vi "list_items.vi"(8 "error in (no error)":errorcluster, 11 "Table in":refnum<class "Table.lvclass">) -> (0 "error out":errorcluster, 2 "items":string[](array[string]), 3 "Table out":refnum<class "Table.lvclass">)   [LabVIEW 2020, in "toml_edit.lvlib" / "Table.lvclass"]
uses:
  Table.lvclass
  Table.lvclass/Table.ctl
  toml_edit.lvlib
  dragon_toml_64.dll
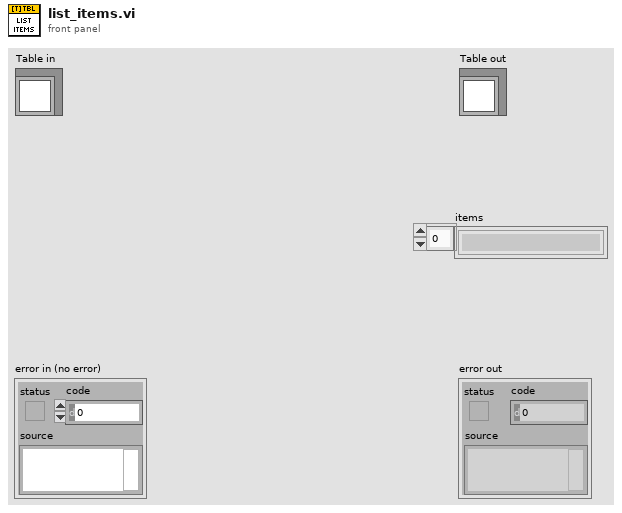
[diagram p1: front panel]
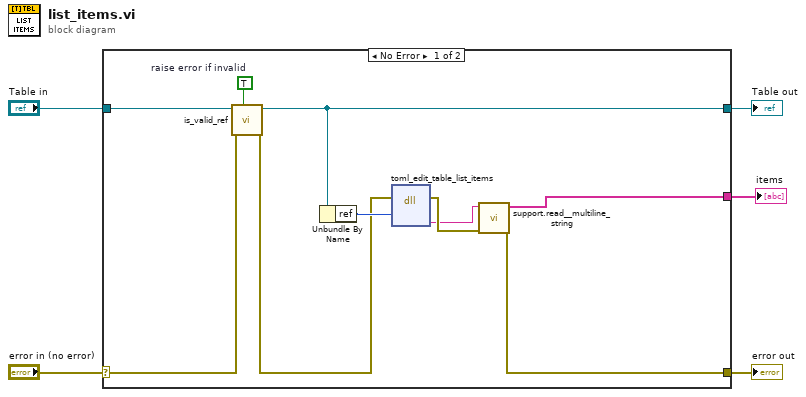
[diagram p0: block diagram]
diagram:
  n1 = case shown="No Error" "error in (no error)" {
    selector: "error in (no error)" -> [w8 w17]
    tunnel: [w13 w17] -> w4
    tunnel: [w11 w16] -> w2
    tunnel: "Table in" -> [w10 w16]
    tunnel: [w12 _] -> w1
    frame No Error {
      w9 = TRUE  # raise error if invalid
      n2 = call-dynamic "is_valid_ref.vi"("raise error if invalid? (False)"=w9, "error in (no error)"=w8, "Table in"=w10) -> ("error out"=w7:errorcluster, "Table out"=w11:refnum<class "Table.lvclass">)  [unwired: 6 in, 1 out]
      n3 = Unbundle By Name(w11) -> ("ref"=w14:u64)
      n4 = dll-call lib="C:/Users/JamesMcNally/Documents/toml-edit-labview/lv_src/dragon_toml_*.dll" fn="toml_edit_table_list_items"(error in=w7, "table_ref"=w14) -> (error out=w15:errorcluster, "item_list"=w6:string)  [unwired: 5 in, 1 out]
      n5 = call "support.read__multiline_string.vi"("error in (no error)"=w15, "table_names"=w6) -> ("error out"=w13:errorcluster, "lines"=w12:string[])  [unwired: 8 in]
    }
    frame Error {
    }
  }
  "error out" <- w4
  "Table out" <- w2
  "items" <- w1
